vi "Otm Mgr Loop.vi"(8 "error in (no error)":errorcluster, 11 "Message Queues":T1) -> (0 "error out":errorcluster)   [LabVIEW 2017]
doc: "Message loop for handling messages pertaining to the acquisition of data from the hardware."
uses:
  <vilib>/Utility/error.llb/Error Cluster From Error Code.vi
  Acquisition/Acquisition.lvlib
  support/Message Queue/Message Queue.lvlib
  Acquisition/Acquisition State.ctl
  support/Message Queue/Enqueue Message (Single).vi
  <vilib>/ErrorRing/Error Ring.xnode
  support/Message Queue/Message Cluster.ctl
  support/Message Queue/All Message Queues.ctl
panel:
  out "运行时间":dbl
  in  "测试时间":dbl=30.0
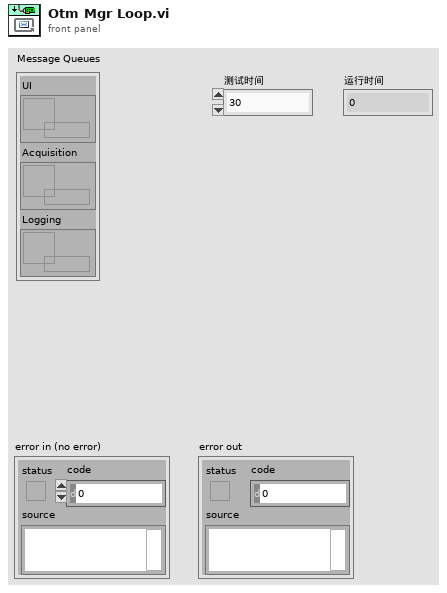
[diagram p1: front panel]
types:
  T1 = typedef "Message Queue.lvlib/All Message Queues.ctl" = cluster{"UI":refnum<queue>, "Acquisition":refnum<queue>, "Logging":refnum<queue>}
  T2 = typedef "Acquisition.lvlib/Acquisition State.ctl" = enum16{"Idle", "Acquiring"}
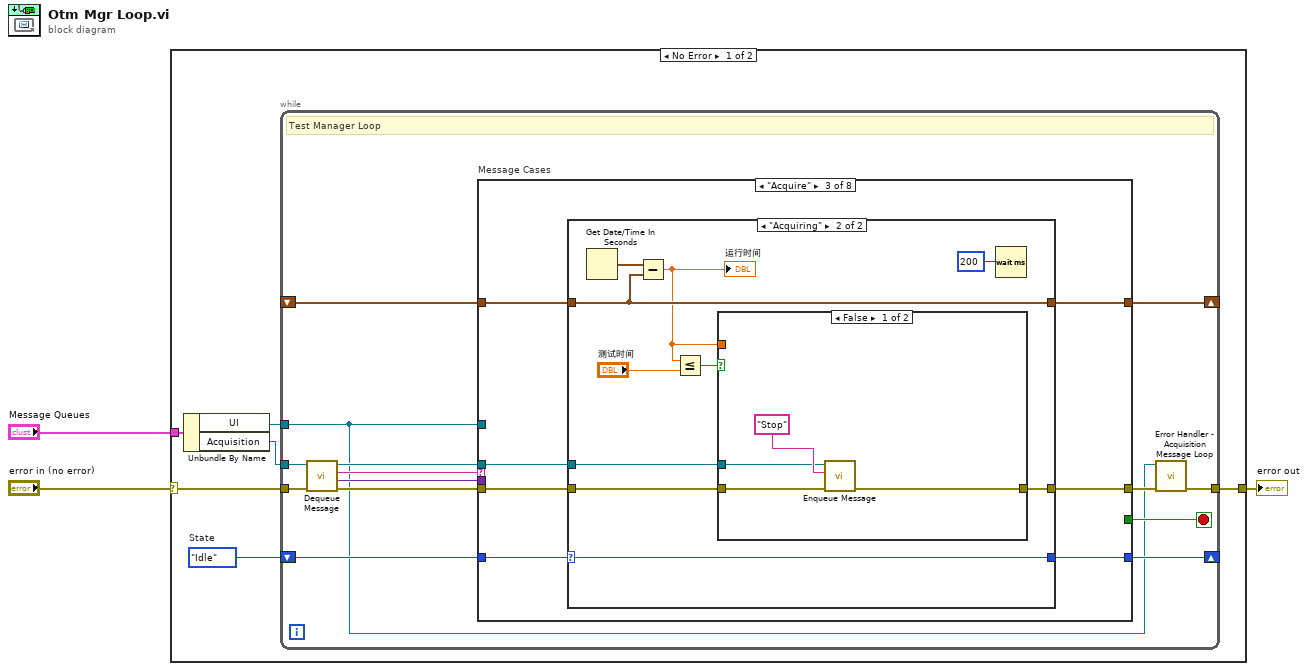
[diagram p0: block diagram]
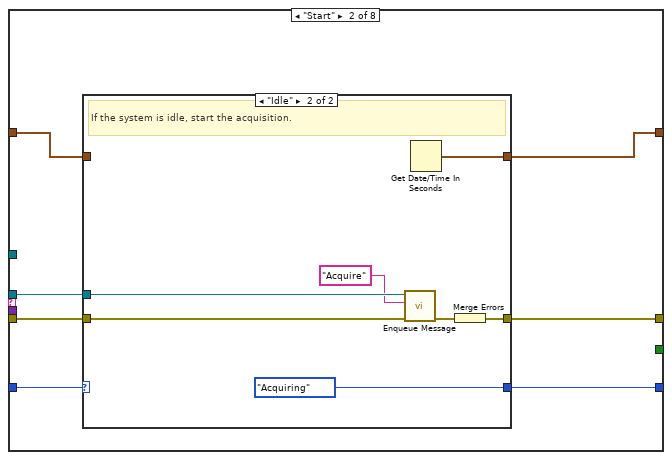
[diagram p3: hidden frame]
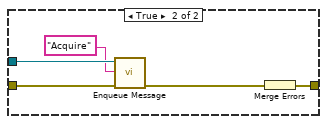
[diagram p6: hidden frame]
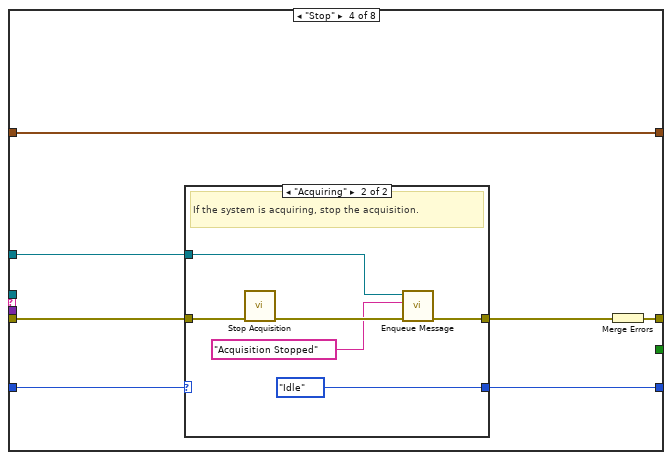
[diagram p7: hidden frame]
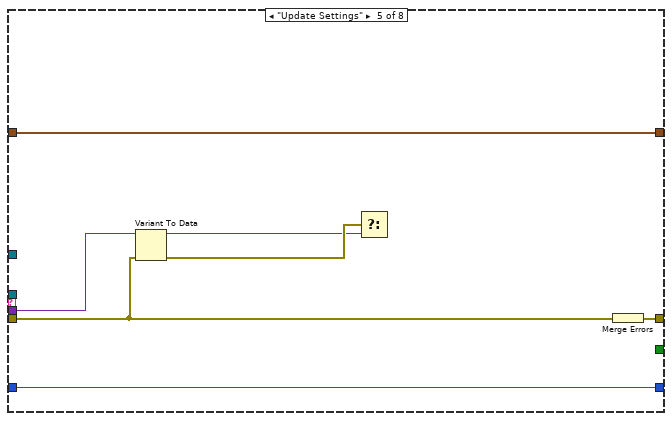
[diagram p9: hidden frame]
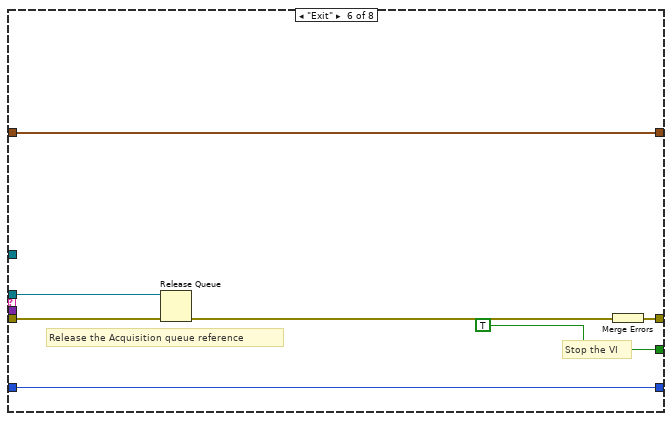
[diagram p10: hidden frame]
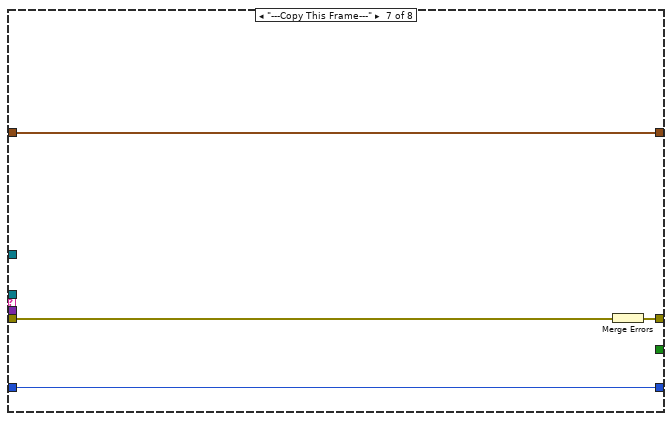
[diagram p11: hidden frame]
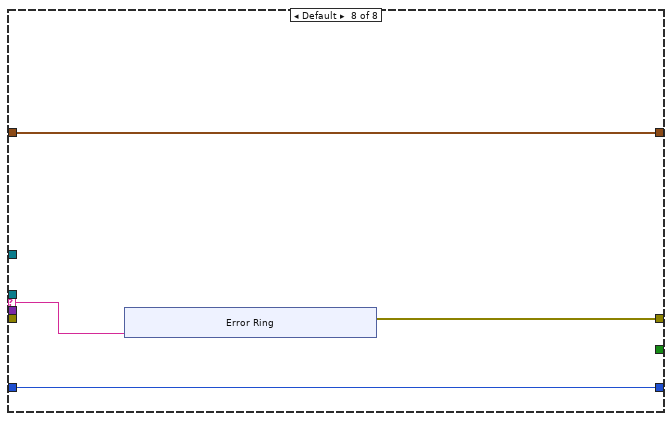
[diagram p12: hidden frame]
diagram:
  n1 = case shown="No Error" "error in (no error)" {
    selector: "error in (no error)" -> [w6 w117]
    tunnel: "Message Queues" -> [w9 _]
    tunnel: [w7 w117] -> w2
    frame No Error {
      w4 = Acquisition_State."Idle"  # State
      n2 = Unbundle By Name(w9) -> ("UI"=w5:refnum<queue>, "Acquisition"=w8:refnum<queue>)
      n3 = while {
        tunnel: w8 -> [w18]
        tunnel: w5 -> [w12]
        shift-right: [w16] -> _
        shift-left: w4 -> [w17]
        tunnel: w6 -> [w22]
        tunnel: [w15] -> w7
        shift-right: [w11] -> _
        shift-left: _ -> [w10]
        stop <- w23 stop-if-true
        # "Test Manager Loop"
        n4 = call "Dequeue Message.vi"("error in (no error)"=w22, "Message Queue"=w18) -> ("error out"=w21:errorcluster, "Message Data"=w19:variant, "Message"=w20:string, "dup Message Queue"=w13:refnum<queue>)  [unwired: 6 in]
        n5 = case "Message Cases" shown="\"Acquire\"" w20 {
          selector: w20 -> [_ _ _ _ _ _ _ w107]
          tunnel: w13 -> [_ w31 w49 _ _ w97 _ _]
          tunnel: w21 -> [w26 w32 w48 w78 w90 w99 w105 _]
          tunnel: [w26 w33 w50 w79 w94 w100 w104 w108] -> w14
          tunnel: [_ _ _ _ _ TRUE _ _] -> w23
          tunnel: w19 -> [_ _ _ _ w93 _ _ _]
          tunnel: w12 -> [_ _ _ w74 _ _ _ _]
          tunnel: w17 -> [w25 w29 w46 w76 w89 w96 w103 w109]
          tunnel: [w25 w30 w47 w75 w89 w96 w103 w109] -> w16
          tunnel: [w24 w28 w44 w73 w88 w95 w102 w106] -> w11
          tunnel: w10 -> [w24 w27 w45 w73 w88 w95 w102 w106]
          frame "Initialize" {
            # "Initialize  - Initialize is currently a no-op.  The hardware initialization takes place in the 'Start' message."
          }
          frame "Start" {
            # "Start - Configure and start the acquisition."
            n6 = case shown="\"Idle\"" w29 {
              selector: w29 -> [w35 _]
              tunnel: [w36 w43] -> w33
              tunnel: w32 -> [w36 w42]
              tunnel: w31 -> [_ w40]
              tunnel: [w35 Acquisition_State."Acquiring" ("Acquisition State")] -> w30
              tunnel: [w34 w37] -> w28
              tunnel: w27 -> [w34 _]
              frame "Acquiring" {
                # "The system is already acquiring. Ignore the \"Start\" message."
              }
              frame "Idle" {
                # "If the system is idle, start the acquisition."
                n7 = call-poly "Enqueue Message.vi"("error in (no error)"=w42, "Message"="Acquire", "Message Queue"=w40) -> ("error out"=w41:errorcluster)  [unwired: 7 in, 1 out]
                n8 = Get Date/Time In Seconds() -> (seconds since 1Jan1904=w37:timestamp)
                n9 = Merge Errors(w41) -> (w43:errorcluster)
              }
            }
          }
          frame "Acquire" {
            # "Acquire - Acquire data from the hardware. Since this is a continuous acquisition, this message will always message itself to run again."
            n10 = case shown="\"Acquiring\"" w46 {
              selector: w46 -> [w52 w61]
              tunnel: [w53 w63] -> w50
              tunnel: w49 -> [_ w62]
              tunnel: w48 -> [w53 w60]
              tunnel: [w52 w61] -> w47
              tunnel: w45 -> [w51 w56]
              tunnel: [w51 w56] -> w44
              frame "Idle" {
                # "Ignore \"Acquire\" messages when the acquisition is idle."
              }
              frame "Acquiring" {
                # "Acquire more data while in the \"Acquiring\" state."
                n11 = Get Date/Time In Seconds() -> (seconds since 1Jan1904=w59:timestamp)
                n12 = Subtract(x=w59, y=w56) -> (x-y=w54:dbl)
                "运行时间" <- w54
                n13 = Less Or Equal?(x=w54, y="测试时间") -> (x <= y?=w57:bool)
                n14 = case shown="False" w57 {
                  tunnel: [w65 w72] -> w63
                  tunnel: w62 -> [w64 w70]
                  tunnel: w60 -> [w66 w68]
                  tunnel: w54 -> [_ _]
                  frame False {
                    n15 = call-poly "Enqueue Message.vi"("error in (no error)"=w66, "Message"="Stop", "Message Queue"=w64) -> ("error out"=w65:errorcluster)  [unwired: 7 in, 1 out]
                  }
                  frame True {
                    n16 = call-poly "Enqueue Message.vi"("error in (no error)"=w68, "Message"="Acquire", "Message Queue"=w70) -> ("error out"=w71:errorcluster)  [unwired: 7 in, 1 out]
                    n17 = Merge Errors(w71) -> (w72:errorcluster)
                  }
                }
                n18 = Wait (ms)(milliseconds to wait=u32 200) -> ()  [unwired: 1 out]
              }
            }
          }
          frame "Stop" {
            # "Stop - Stop the Acquisition."
            n19 = case shown="\"Acquiring\"" w76 {
              selector: w76 -> [w80 _]
              tunnel: w78 -> [w81 w87]
              tunnel: [w81 w84] -> w77
              tunnel: [w80 Acquisition_State."Idle" ("State")] -> w75
              tunnel: w74 -> [_ w83]
              frame "Idle" {
                # "The system is already idle. Ignore the \"Stop\" message."
              }
              frame "Acquiring" {
                # "If the system is acquiring, stop the acquisition."
                n20 = call "Stop Acquisition.vi"("error in (no error)"=w87) -> ("error out"=w86:errorcluster)  [unwired: 10 in]
                n21 = call-poly "Enqueue Message.vi"("error in (no error)"=w86, "Message"="Acquisition Stopped", "Message Queue"=w83) -> ("error out"=w84:errorcluster)  [unwired: 7 in, 1 out]
              }
            }
            n22 = Merge Errors(w77) -> (w79:errorcluster)
          }
          frame "Update Settings" {
            # "New settings are available, update the current ones stored in the shift register with the settings sent as part of the message"
            n23 = Variant To Data(error in=w90, Variant=w93) -> (data=w91:variant, error out=w92:errorcluster)  [unwired: 1 in]
            n24 = Select(s=w92, f=w91) -> ()  [unwired: 1 in, 1 out]
            n25 = Merge Errors(w90) -> (w94:errorcluster)
          }
          frame "Exit" {
            # "Release the Acquisition queue reference"
            # "Stop the VI"
            # "Exit - Send the Exit message to the UI Message Handler."
            n26 = Release Queue(queue=w97, error in (no error)=w99) -> (error out=w98:errorcluster)  [unwired: 1 in, 2 out]
            n27 = Merge Errors(w98) -> (w100:errorcluster)
          }
          frame "---Copy This Frame---" {
            # "Duplicate this frame when creating new messages.  Change this comment in the duplicated frame to describe this message."
            n28 = Merge Errors(w105) -> (w104:errorcluster)
          }
          frame Default {
            # "'Default' case only runs if there is a message that isn't defined in any of the other cases.  Output a programming error."
            n29 = xnode "Error Ring"("parameter 0"=w107) -> ("error out"=w108:errorcluster)
          }
        }
        n30 = call "Error Handler - Acquisition Message Loop.vi"("error in (no error)"=w14, "Message Queue"=w12) -> ("dup error in"=w15:errorcluster)  [unwired: 8 in, 1 out]
      }
    }
    frame Error {
    }
  }
  "error out" <- w2
